vi "MeasHarmSelect.vi"(7 "xFund":dbl, 9 "yMultiplier":dbl, 10 "yMultiplier":string) -> (1 "X x Y":dbl, 2 "Boolean":bool)   [LabVIEW 2018]
panel:
  # "Makes decision based on yMultiplier\nIF O = fALSE\nIF"
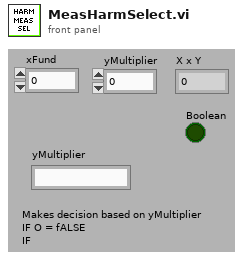
[diagram p1: front panel]
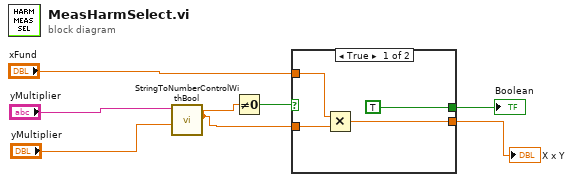
[diagram p0: block diagram]
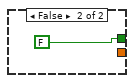
[diagram p2: hidden frame]
diagram:
  n1 = call "StringToNumberControlWithBool.vi"("Numeric In"="yMultiplier", "String In"="yMultiplier") -> ("Number Out"=w1:dbl)  [unwired: 6 in, 1 out]
  n2 = Not Equal To 0?(x=w1) -> (x != 0?=w2:bool)
  n3 = case shown="True" w2 {
    tunnel: [TRUE FALSE] -> w7
    tunnel: "xFund" -> [w10 _]
    tunnel: [w9 _] -> w3
    tunnel: w1 -> [w8 _]
    frame True {
      n4 = Multiply(x=w10, y=w8) -> (x*y=w9:dbl)
    }
    frame False {
    }
  }
  "Boolean" <- w7
  "X x Y" <- w3
